vi "Dictionary Has Key__ogtk.vi"(8 "error in (no error)":errorcluster, 10 "key":variant, 11 "dictionary":T1) -> (0 "error out":errorcluster, 2 "Has Key?":bool, 3 "dictionary out":T1)   [LabVIEW 2011]
doc: "Determines if the supplied key is present in the dictionary."
uses:
  Dictionary Object RefNum__ogtk.ctl
  Dictionary Object RefNum - Enum__ogtk.ctl
panel:
  # "Dictionary Has Key.vi\n\nDetermines if the supplied key is present in the dictionary.\n\nPlease visit http://www.OpenG.org to learn about the\nOpen Source LabVIEW software movement.\n\nNOTICE -- YOU MUST LEAVE THIS NOTICE IN PLACE.  PER THE TERMS OF THE LICENSE BELOW, YOU MAY SUBLICENSE THIS SOFTWARE \nIN ANY WAY THAT DOES NOT CONFLICT WITH THIS LICENSE.\n\n### BSD License (http://www.opensource.org/licenses/bsd-license.php) Begin ###\n \nCopyright (c) 2005, Jim Kring <jim@jimkring.com>\n\nAll rights reserved.\n\nRedistribution and use in source and binary forms, with or without modification, are permitted provided that the following conditions are met:\n\n    * Redistributions of source code must retain the above copyright notice, this list of conditions and the following disclaimer.\n    * Redistributions in binary form must reproduce the above copyright notice, this list of conditions and the following disclaimer in the \n       documentation and/or other materials provided with the distribution.\n    * Neither the name of SciWare, James Kring, Inc., nor the names of its contributors may be used to endorse or promote products derived \n       from this software without specific prior written permission.\n\nTHIS SOFTWARE IS PROVIDED BY THE COPYRIGHT HOLDERS AND CONTRIBUTORS \"AS IS\" AND ANY EXPRESS OR IMPLIED WARRANTIES, \nINCLUDING, BUT NOT LIMITED TO, THE IMPLIED WARRANTIES OF MERCHANTABILITY AND FITNESS FOR A PARTICULAR PURPOSE ARE \nDISCLAIMED. IN NO EVENT SHALL THE COPYRIGHT OWNER OR CONTRIBUTORS BE LIABLE FOR ANY DIRECT, INDIRECT, INCIDENTAL,\n SPECIAL, EXEMPLARY, OR CONSEQUENTIAL DAMAGES (INCLUDING, BUT NOT LIMITED TO, PROCUREMENT OF SUBSTITUTE GOODS OR \nSERVICES; LOSS OF USE, DATA, OR PROFITS; OR BUSINESS INTERRUPTION) HOWEVER CAUSED AND ON ANY THEORY OF LIABILITY, \nWHETHER IN CONTRACT, STRICT LIABILITY, OR TORT (INCLUDING NEGLIGENCE OR OTHERWISE) ARISING IN ANY WAY OUT OF THE USE \nOF THIS SOFTWARE, EVEN IF ADVISED OF THE POSSIBILITY OF SUCH DAMAGE.\n\n### BSD License End ###"
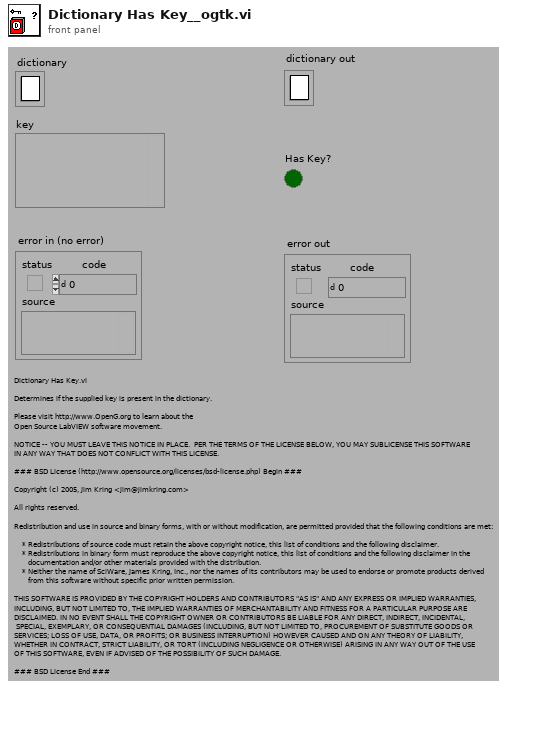
[diagram p1: front panel]
types:
  T1 = typedef "Dictionary Object RefNum__ogtk.ctl" = refnum<k1>
  T2 = typedef "Dictionary Data__ogtk.ctl" = cluster{"keys":variant[], "values":variant[]}
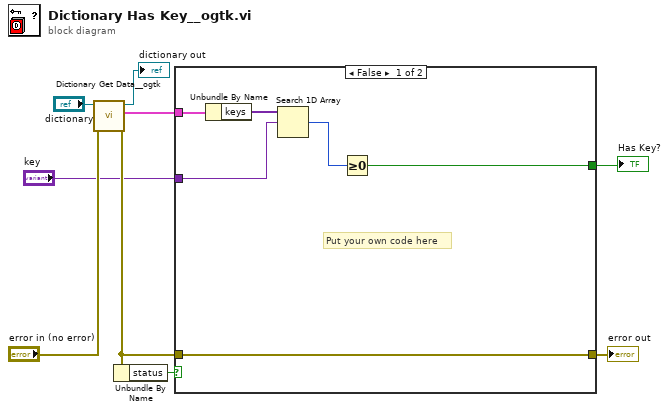
[diagram p0: block diagram]
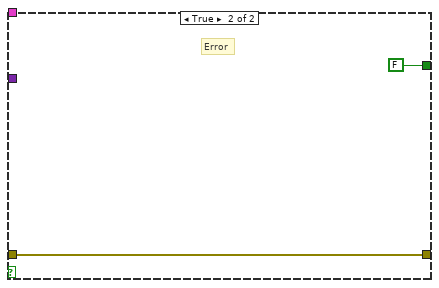
[diagram p2: hidden frame]
diagram:
  n1 = call "Dictionary Get Data__ogtk.vi"("error in (no error)"="error in (no error)", "Object RefNum"="dictionary") -> ("error out"=w5:errorcluster, "Data out"=w7:T2, "Dup Object RefNum"=→"dictionary out":T1)  [unwired: 7 in]
  n2 = Unbundle By Name(w5) -> ("status"=w9:bool)
  n3 = case shown="False" w9 {
    tunnel: w5 -> [w14 w17]
    tunnel: [w14 w17] -> w8
    tunnel: w7 -> [w15 _]
    tunnel: "key" -> [w12 _]
    tunnel: [w11 FALSE] -> w1
    frame False {
      # "Put your own code here"
      n4 = Unbundle By Name(w15) -> ("keys"=w13:variant[])
      n5 = Search 1D Array(1D array=w13, element=w12) -> (index of element=w10:i32)  [unwired: 1 in]
      n6 = Greater Or Equal To 0?(x=w10) -> (x >= 0?=w11:bool)
    }
    frame True {
      # "Error"
    }
  }
  "error out" <- w8
  "Has Key?" <- w1
